vi "Init Bfr Rx - Create Buffer.vi"(8 "error in (no error)":errorcluster, 11 "Rx Loop Data in":T1 {"Buffer Resources"."Data Buffer" format="%016x"; "Buffer Option Support"."Ping Pong Buffer"."Active Buffer Ref" format="%016x"; "Buffer Option Support"."Cached Buffer"."Cache Buffer" format="%016x"}) -> (0 "error out":errorcluster, 3 "Rx Loop Data out":T1 {"Buffer Resources"."Data Buffer" format="%016x"; "Buffer Option Support"."Ping Pong Buffer"."Active Buffer Ref" format="%016x"; "Buffer Option Support"."Cached Buffer"."Cache Buffer" format="%016x"})   [LabVIEW 2019, in "UDP-Custom-Device Engine.lvlib"]
uses:
  UDP-Custom-Device Engine.lvlib
  Types/Engine - Buffered Rx Loop Data.ctl
  Types/Engine - General Resources.ctl
  <vilib>/NI VeriStand/VeriStand Data/Typedefs/Typedefs.Data Types.ctl
  Shared/Types/Shared - Duplex Settings.ctl
  Shared/Types/Shared - Header Details.ctl
  Shared/Types/Shared - Custom Header.ctl
  Types/Engine - Buffer Resources.ctl
  Shared/Types/Shared - Pointer Encoding.ctl
  Types/Engine - Rx Runtime Resources.ctl
  Types/Engine - Execution Config.ctl
  Shared/Types/Shared - Thread Management.ctl
  Types/Engine - Rx New Data Options Support.ctl
  Shared/Types/Shared - New Data Options.ctl
  Types/Engine - Buffered Rx Buffer Option Support.ctl
  Shared/Types/Shared - Receive Buffer Options.ctl
  Types/Engine - Buffered Rx Circular Buffer.ctl
  Types/Engine - Buffered Rx Cached Buffer.ctl
  Types/Engine - Buffered Rx Ping Pong Buffer.ctl
  Types/Engine - Buffered Rx Active Buffer.ctl
  Types/Engine - Buffered Rx Channel Refs.ctl
  <vilib>/NI/NIVS Inline Async API/_Data Access Engine/Data Access Engine/Types/Write.DVR.ctl
  <vilib>/NI/NIVS Inline Async API/_Data Access Engine/Access Type Classes/Write/Write.lvclass
  <vilib>/NI/NIVS Inline Async API/_Data Access Engine/Data Access Engine/Types/Read.DVR.ctl
  <vilib>/NI/NIVS Inline Async API/_Data Access Engine/Access Type Classes/Read/Read.lvclass
  Types/Engine - Buffered Rx Ping Pong Channels.ctl
  Types/Engine - Debug Resources.ctl
  <vilib>/NI/NIVS Inline Async API/_Data Access Engine/Access Type Classes/Write/Write.lvclass/Write.ctl
  <vilib>/NI VeriStand/VeriStand Data/Pointer Operations/Pointer.Write (1D U8).vi
  <vilib>/NI/NIVS Inline Async API/_Data Access Engine/Data Access Engine/Methods/Write.Data.vi
  <vilib>/NI/NIVS Inline Async API/_Data Access Engine/Access Type Classes/Write/Write.ProcessData.vi
  <vilib>/NI VeriStand/VeriStand Data/Pointer Operations/Pointer.Write (U8).vi
  <vilib>/NI VeriStand/VeriStand Data/Pointer Operations/Pointer.Write (U16).vi
  <vilib>/NI VeriStand/VeriStand Data/VeriStand Data.lvlib
  <vilib>/NI/NIVS Inline Async API/_Data Access Engine/Data Access Engine/Data Access Engine.lvclass
  Shared/UDP-Custom-Device Shared.lvlib
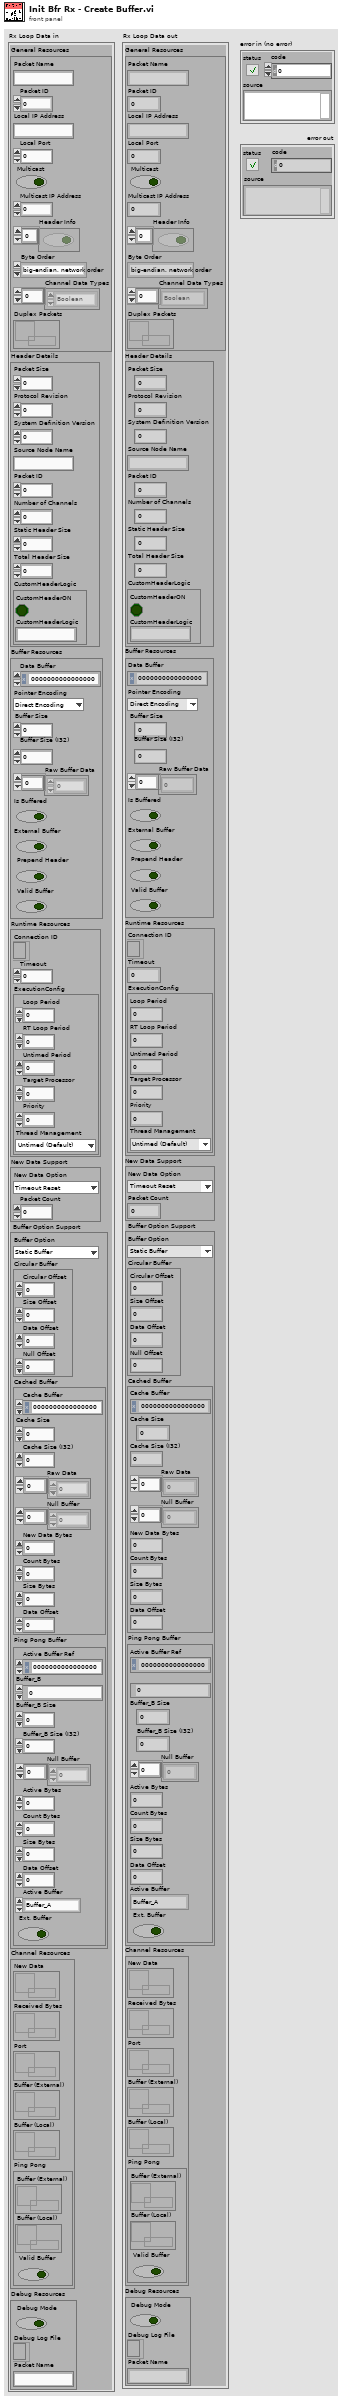
[diagram p1: front panel]
types:
  T1 = typedef "UDP-Custom-Device Engine.lvlib/Engine - Buffered Rx Loop Data.ctl" = cluster{"General Resources":T2, "Header Details":T4, "Buffer Resources":T6, "Runtime Resources":T8, "New Data Support":T11, "Buffer Option Support":T13, "Channel Resources":T19, "Debug Resources":T23}
  T2 = typedef "UDP-Custom-Device Engine.lvlib/Engine - General Resources.ctl" = cluster{"Packet Name":string, "Packet ID":i32, "Local IP Address":string, "Local Port":i32, "Multicast":bool, "Multicast IP Address":u32, "Header Info":bool[], "Byte Order":enum16{"big-endian, network order", "native, host order", "little-endian"}, "Channel Data Types":T3[], "Duplex Packets":refnum<data-value>}
  T3 = typedef "VeriStand Data.lvlib/Typedefs.Data Types.ctl" = enum16{"Boolean", "Single", "Double", "I8", "I16", "I32", "I64", "U8", "U16", "U32", "U64"}
  T4 = typedef "UDP-Custom-Device Shared.lvlib/Shared - Header Details.ctl" = cluster{"Packet Size":u16, "Protocol Revision":u8, "System Definition Version":u64, "Source Node Name":string, "Packet ID":u32, "Number of Channels":u32, "Static Header Size":u16, "Total Header Size":u16, "CustomHeaderLogic":T5}
  T5 = typedef "UDP-Custom-Device Shared.lvlib/Shared - Custom Header.ctl" = cluster{"CustomHeaderON":bool, "CustomHeaderLogic":string}
  T6 = typedef "UDP-Custom-Device Engine.lvlib/Engine - Buffer Resources.ctl" = cluster{"Data Buffer":u64, "Pointer Encoding":T7, "Buffer Size":u64, "Buffer Size (I32)":i32, "Raw Buffer Data":u8[], "Is Buffered":bool, "External Buffer":bool, "Prepend Header":bool, "Valid Buffer":bool}
  T7 = typedef "UDP-Custom-Device Shared.lvlib/Shared - Pointer Encoding.ctl" = enum16{"Direct Encoding", "Conversion Encoding"}
  T8 = typedef "UDP-Custom-Device Engine.lvlib/Engine - Rx Runtime Resources.ctl" = cluster{"Connection ID":refnum<k16>, "Timeout":i32, "ExecutionConfig":T9}
  T9 = typedef "UDP-Custom-Device Engine.lvlib/Engine - Execution Config.ctl" = cluster{"Loop Period":i64, "RT Loop Period":i64, "Untimed Period":u32, "Target Processor":i32, "Priority":i32, "Thread Management":T10}
  T10 = typedef "UDP-Custom-Device Shared.lvlib/Shared - Thread Management.ctl" = enum16{"Untimed (Default)", "Timed (High Priority)"}
  T11 = typedef "UDP-Custom-Device Engine.lvlib/Engine - Rx New Data Options Support.ctl" = cluster{"New Data Option":T12, "Packet Count":dbl}
  T12 = typedef "UDP-Custom-Device Shared.lvlib/Shared - New Data Options.ctl" = enum16{"Timeout Reset", "Counter"}
  T13 = typedef "UDP-Custom-Device Engine.lvlib/Engine - Buffered Rx Buffer Option Support.ctl" = cluster{"Buffer Option":T14, "Circular Buffer":T15, "Cached Buffer":T16, "Ping Pong Buffer":T17}
  T14 = typedef "UDP-Custom-Device Shared.lvlib/Shared - Receive Buffer Options.ctl" = enum16{"Static Buffer", "Circular Buffer", "Circular Buffer + Size", "Internal Cache", "Internal Cache + Size", "Ping Pong", "Ping Pong + Size"}
  T15 = typedef "UDP-Custom-Device Engine.lvlib/Engine - Buffered Rx Circular Buffer.ctl" = cluster{"Circular Offset":u64, "Size Offset":u64, "Data Offset":u64, "Null Offset":u64}
  T16 = typedef "UDP-Custom-Device Engine.lvlib/Engine - Buffered Rx Cached Buffer.ctl" = cluster{"Cache Buffer":u64, "Cache Size":u64, "Cache Size (I32)":i32, "Raw Data":u8[], "Null Buffer":u8[], "New Data Bytes":u64, "Count Bytes":u64, "Size Bytes":u64, "Data Offset":u64}
  T17 = typedef "UDP-Custom-Device Engine.lvlib/Engine - Buffered Rx Ping Pong Buffer.ctl" = cluster{"Active Buffer Ref":u64, "Buffer_B":u64, "Buffer_B Size":u64, "Buffer_B Size (I32)":i32, "Null Buffer":u8[], "Active Bytes":u64, "Count Bytes":u64, "Size Bytes":u64, "Data Offset":u64, "Active Buffer":T18, "Ext. Buffer":bool}
  T18 = typedef "UDP-Custom-Device Engine.lvlib/Engine - Buffered Rx Active Buffer.ctl" = enum16{"Buffer_A", "Buffer_B"}
  T19 = typedef "UDP-Custom-Device Engine.lvlib/Engine - Buffered Rx Channel Refs.ctl" = cluster{"New Data":T20, "Received Bytes":T20, "Port":T20, "Buffer (External)":T21, "Buffer (Local)":T20, "Ping Pong":T22}
  T20 = typedef "Data Access Engine.lvlib/Data Access Engine.lvclass/Write.DVR.ctl" = refnum<data-value>
  T21 = typedef "Data Access Engine.lvlib/Data Access Engine.lvclass/Read.DVR.ctl" = refnum<data-value>
  T22 = typedef "UDP-Custom-Device Engine.lvlib/Engine - Buffered Rx Ping Pong Channels.ctl" = cluster{"Buffer (External)":T21, "Buffer (Local)":T20, "Valid Buffer":bool}
  T23 = typedef "UDP-Custom-Device Engine.lvlib/Engine - Debug Resources.ctl" = cluster{"Debug Mode":bool, "Debug Log File":refnum<file>, "Packet Name":string}
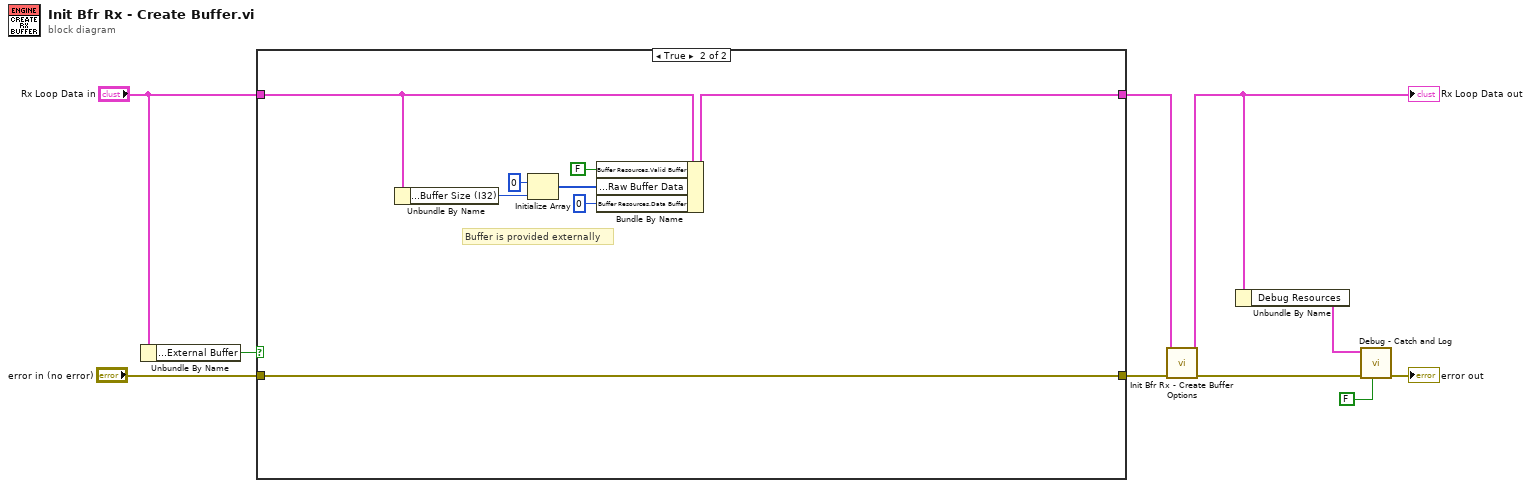
[diagram p0: block diagram]
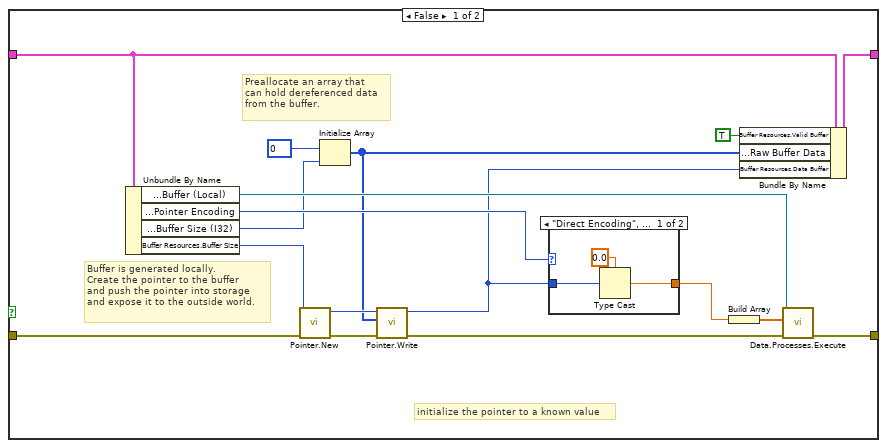
[diagram p2: hidden frame]
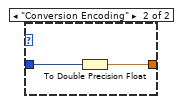
[diagram p3: hidden frame]
diagram:
  n1 = Unbundle By Name("Rx Loop Data in") -> ("Buffer Resources.External Buffer"=w8:bool)
  n2 = case shown="True" w8 {
    tunnel: "error in (no error)" -> [w27 w40]
    tunnel: [w22 w40] -> w3
    tunnel: "Rx Loop Data in" -> [w26 w35]
    tunnel: [w25 w34] -> w1
    frame False {
      # "initialize the pointer to a known value"
      # "Preallocate an array that\ncan hold dereferenced data\nfrom the buffer."
      # "Buffer is generated locally.\nCreate the pointer to the buffer\nand push the pointer into storage\nand expose it to the outside world."
      n3 = Unbundle By Name(w26) -> ("Channel Resources.Buffer (Local)"=w24:T20, "Buffer Resources.Pointer Encoding"=w17:T7, "Buffer Resources.Buffer Size (I32)"=w11:i32, "Buffer Resources.Buffer Size"=w12:u64)
      n4 = call <vilib>:"Pointer.New.vi"("error in (no error)"=w27, "size in bytes"=w12) -> ("error out"=w20:errorcluster, "pointer"=w19:u64)  [unwired: 8 in]
      n5 = Initialize Array(u8 0, w11) -> (w13:u8[])
      n6 = call-poly <vilib>:"Pointer.Write.vi"("error in (no error)"=w20, "values"=w13, "pointer in"=w19) -> ("error out"=w14:errorcluster, "pointer out"=w15:u64)  [unwired: 6 in, 1 out]
      n7 = case shown="\"Direct Encoding\", Default" w17 {
        tunnel: w15 -> [w30 w32]
        tunnel: [w29 w31] -> w18
        frame "Direct Encoding", Default {
          n8 = Type Cast(type=0.0, x=w30) -> (*(type *) &x=w29:dbl)
        }
        frame "Conversion Encoding" {
          n9 = To Double Precision Float(number=w32) -> (double precision float=w31:dbl)
        }
      }
      n10 = Build Array(w18) -> (w23:dbl[])
      n11 = Bundle By Name(cluster=w26, "Buffer Resources.Valid Buffer"=TRUE ("Valid Buffer"), "Buffer Resources.Raw Buffer Data"=w13, "Buffer Resources.Data Buffer"=w15) -> (w25:T1)
      n12 = call-poly <vilib>:"Data.Processes.Execute.vi"("error in (no error)"=w14, "Values"=w23, "Ref"=w24) -> ("error out"=w22:errorcluster)  [unwired: 8 in]
    }
    frame True {
      # "Buffer is provided externally"
      n13 = Unbundle By Name(w35) -> ("Buffer Resources.Buffer Size (I32)"=w38:i32)
      n14 = Initialize Array(u8 0, w38) -> (w33:u8[])
      n15 = Bundle By Name(cluster=w35, "Buffer Resources.Valid Buffer"=FALSE ("Valid Buffer"), "Buffer Resources.Raw Buffer Data"=w33, "Buffer Resources.Data Buffer"=u64 0 ("Data Buffer")) -> (w34:T1)
    }
  }
  n16 = call "Init Bfr Rx - Create Buffer Options.vi"("error in (no error)"=w3, "Rx Loop Data in"=w1) -> ("error out"=w4:errorcluster, "Rx Loop Data out"=w2:T1)  [unwired: 8 in]
  "Rx Loop Data out" <- w2
  n17 = Unbundle By Name(w2) -> ("Debug Resources"=w6:T23)
  n18 = call "Debug - Catch and Log.vi"("Clear Error?"=FALSE, "error in (no error)"=w4, "Debug Resources"=w6) -> ("error out"=→"error out":errorcluster)  [unwired: 8 in]
